vi "Server_Save.vi"(8 "error in (no error)":errorcluster, 9 "Code":string, 10 "Name":string="file.py", 11 "Server":path) -> (0 "error out":errorcluster)   [LabVIEW 2020]
panel:
  out "length":i32
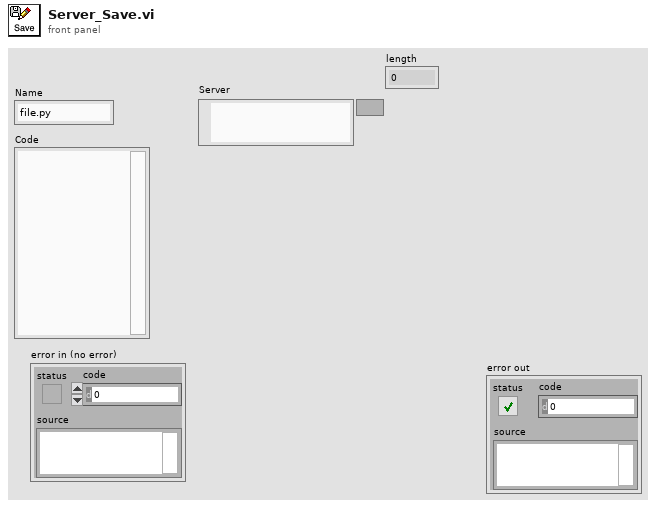
[diagram p1: front panel]
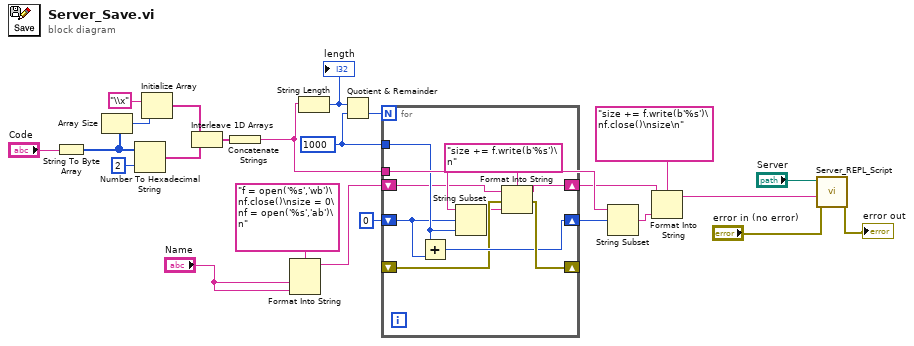
[diagram p0: block diagram]
diagram:
  w10 = 1000 ("y")
  n1 = String To Byte Array(string="Code") -> (unsigned byte array=w22:u8[])
  n2 = Array Size(array=w22) -> (size(s)=w21:i32)
  n3 = Number To Hexadecimal String(1:i16 2 ("width (-)"), 2:w22) -> (0:w19:string[])
  n4 = Initialize Array("\\x", w21) -> (w20:string[])
  n5 = Interleave 1D Arrays(w20, w19) -> (w18:string[])
  n6 = Concatenate Strings(w18) -> (w8:string)
  n7 = Format Into String(format string="f = open('%s','wb')\nf.close()\nsize = 0\nf = open('%s','ab')\n", "Name", "Name") -> (resulting string=w6:string)  [unwired: 2 in, 1 out]
  n8 = String Length(string=w8) -> (length=w13:i32)
  "length" <- w13
  n9 = Quotient & Remainder(x=w13, y=w10) -> (floor(x/y)=w12:i32)  [unwired: 1 out]
  n10 = for {
    N: w12 -> [_]
    tunnel: w8 -> [w33]
    shift-right: [w34] -> _
    shift-left: _ -> [w29]
    shift-right: [w30] -> w9
    shift-left: 0 ("y") -> [w31]
    tunnel: w10 -> [w32]
    shift-right: [w27] -> w2
    shift-left: w6 -> [w25]
    n11 = Add(x=w32, y=w31) -> (x+y=w30:i32)
    n12 = String Subset(string=w33, offset (0)=w31, length (rest)=w32) -> (substring=w28:string)
    n13 = Format Into String(format string="size += f.write(b'%s')\n", initial string=w25, error in=w29, w28) -> (resulting string=w27:string, error out=w34:errorcluster)
  }
  n14 = String Subset(string=w8, offset (0)=w9) -> (substring=w4:string)  [unwired: 1 in]
  n15 = Format Into String(format string="size += f.write(b'%s')\nf.close()\nsize\n", initial string=w2, w4) -> (resulting string=w1:string)  [unwired: 1 in, 1 out]
  n16 = call "Server_REPL_Script.vi"("error in (no error)"="error in (no error)", "Code"=w1, "Server"="Server") -> ("error out"=→"error out":errorcluster)  [unwired: 8 in]
